vi "LVClasse_SurfaceFloat Write SurfaceFloat.vi"(8 "error in (no error)":errorcluster, 10 "SurfaceFloat":T1, 11 "SurfaceFloat in":refnum<class "SurfaceFloat.lvclass">) -> (0 "error out":errorcluster, 3 "SurfaceFloat out":refnum<class "SurfaceFloat.lvclass">)   [LabVIEW 2020, in "SurfaceFloat.lvclass"]
uses:
  SurfaceFloat.lvclass
  ClassID.ctl
  Handle creation.ctl
  SurfaceFloat.lvclass/SurfaceFloat.ctl
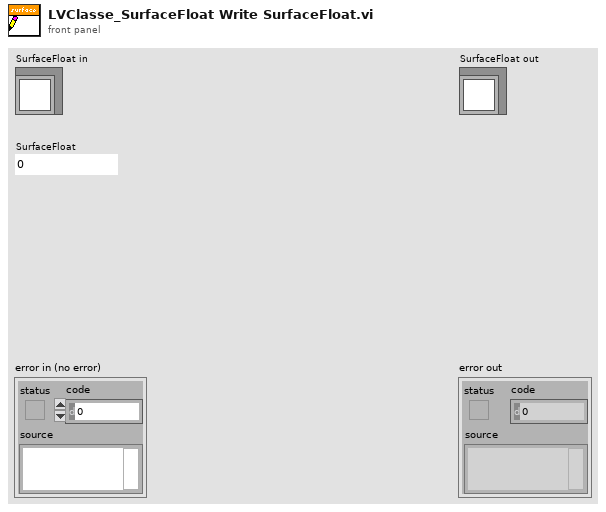
[diagram p1: front panel]
types:
  T1 = typedef "ClassID.ctl" = i64
  T2 = typedef "Handle creation.ctl" = enum16{"By ctor", "By write function"}
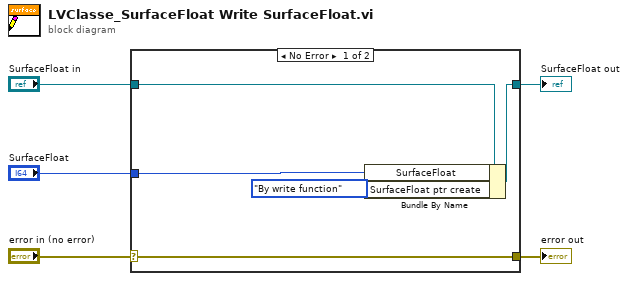
[diagram p0: block diagram]
diagram:
  n1 = case shown="No Error" "error in (no error)" {
    selector: "error in (no error)" -> [w10 w11]
    tunnel: [w10 w11] -> w4
    tunnel: [w8 w12] -> w2
    tunnel: "SurfaceFloat in" -> [w9 w12]
    tunnel: "SurfaceFloat" -> [w7 _]
    frame No Error {
      n2 = Bundle By Name(cluster=w9, "SurfaceFloat"=w7, "SurfaceFloat ptr create"=Handle_creation."By write function") -> (w8:refnum<class "SurfaceFloat.lvclass">)
    }
    frame Error {
    }
  }
  "error out" <- w4
  "SurfaceFloat out" <- w2
